vi "FPGA_AIReadConfig.vi"(8 "error in (no error)":errorcluster, 11 "AI Reference":T1) -> (0 "error out":errorcluster, 1 "Convert Rate":u32, 2 "Scan Size":u8, 3 "AI Reference":T1)   [LabVIEW 2017]
uses:
  <vilib>/Rock Robotics/SystemInterfaces/AI/FPGA_AIDevRef.ctl
  <vilib>/Rock Robotics/SystemInterfaces/System/FPGA_SystemFPGA Ref Global.vi
  <vilib>/Utility/error.llb/Error Cluster From Error Code.vi
  <vilib>/rvi/errors/niLvFpgaAdjustHostInterfaceError.vi
  <vilib>/rvi/interface/nirviReadWriteControl/nirviReadWriteControl.xnode
  <vilib>/Rock Robotics/SystemInterfaces/System/FPGA_SystemFRC FPGA Ref.ctl
  NiFpgaLv.dll
  <vilib>/rvi/interface/Simulation/niFpgaSimulationCallBeginRW.vi
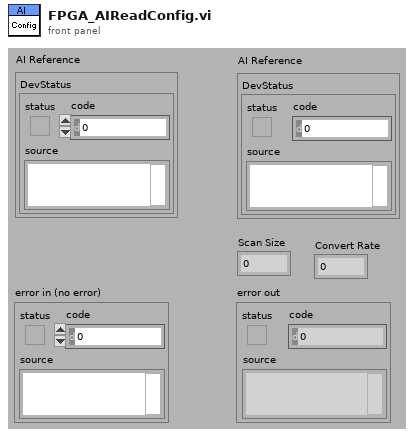
[diagram p1: front panel]
types:
  T1 = typedef "FPGA_AIDevRef.ctl" = cluster{"DevStatus":errorcluster}
  T2 = typedef "FPGA_SystemFRC FPGA Ref.ctl" = refnum<k20>
  T3 = cluster{"ScanSize":fxp<+,3,3>, "ConvertRate":fxp<+,26,26>}
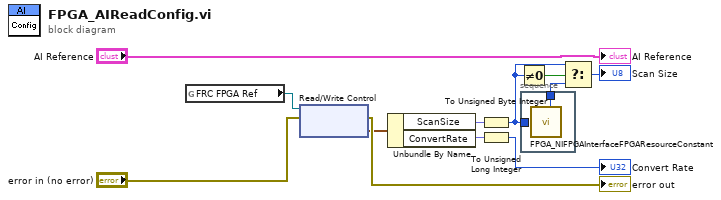
[diagram p0: block diagram]
diagram:
  n1 = global read "FPGA_SystemFPGA Ref Global.vi" "FRC FPGA Ref"() -> (w3:T2)
  n2 = xnode "Read/Write Control"("FPGA VI Reference In"=w3, "error in"="error in (no error)") -> ("error out"=→"error out":errorcluster, "AI.Config"=w1:T3)  [unwired: 1 out]
  n3 = Unbundle By Name(w1) -> ("ScanSize"=w7:fxp<+,3,3>, "ConvertRate"=w6:fxp<+,26,26>)
  n4 = To Unsigned Byte Integer(number=w7) -> (unsigned 8bit integer=w2:u8)
  n5 = To Unsigned Long Integer(number=w6) -> (unsigned 32bit integer=→"Convert Rate":u32)
  n6 = Not Equal To 0?(x=w2) -> (x != 0?=w5:bool)
  n7 = stacked-sequence {
    tunnel: [w13] -> w4
    tunnel: w2 -> [_]
    frame #0 {
      n8 = call <vilib>:"FPGA_NIFPGAInterfaceFPGAResourceConstant.vi"() -> ("NumberOfAIChannels"=w13:u8)  [unwired: 11 out]
    }
  }
  n9 = Select(t=w2, s=w5, f=w4) -> (s? t:f=→"Scan Size":u8)
  "AI Reference" <- "AI Reference"
